vi "Write extended.vi"(8 "error in (no error)":errorcluster, 10 "extended":map{string, string}(c390), 11 "file attributes in":refnum<class "File Attributes.lvclass">) -> (0 "error out":errorcluster, 3 "file attributes out":refnum<class "File Attributes.lvclass">)   [LabVIEW 2020, in "NI_SFTP.lvlib" / "File Attributes.lvclass"]
doc: "Writes extended file attributes into the specified File Attributes object. Any existing extended attributes are replaced. The nature of these attributes is server-dependent."
uses:
  <vilib>/net/SFTP/File Attributes/File Attributes.lvclass
  <vilib>/net/SFTP/File Attributes/File Attributes.lvclass/File Attributes.ctl
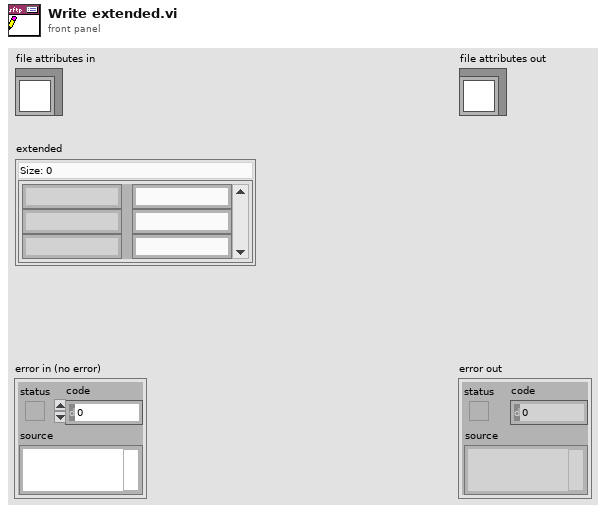
[diagram p1: front panel]
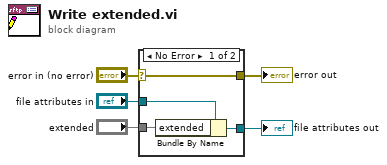
[diagram p0: block diagram]
diagram:
  n1 = case shown="No Error" "error in (no error)" {
    selector: "error in (no error)" -> [w9 w10]
    tunnel: [w9 w10] -> w4
    tunnel: [w7 w11] -> w2
    tunnel: "file attributes in" -> [w8 w11]
    tunnel: "extended" -> [w6 _]
    frame No Error {
      n2 = Bundle By Name(cluster=w8, "extended"=w6) -> (w7:refnum<class "File Attributes.lvclass">)
    }
    frame Error {
    }
  }
  "error out" <- w4
  "file attributes out" <- w2
